vi "Teleop.vi"(10 "Match Info":T1={"Autonomous Elapsed Seconds"=0.0, "TeleOp Elapsed Seconds"=0.0, "Disabled Elapsed Seconds"=0.0, "Visited Autonomous"=FALSE, "Visited TeleOp"=FALSE, "Visited Disabled"=FALSE, "Autonomous Settings"={"Autonomous Style"=enum."Independent", "VI Refnum"=refnum}}, 11 "Call Context":T2) -> ()   [LabVIEW 2020]
doc: "This VI is called for each TeleOp packet received from the DS where the robot is not disabled. It is often used to read from the joysticks and update I/O or to update setpoints for timed control loops. It should complete and return within 20 milliseconds or it may miss DS packets."
uses:
  <vilib>/Rock Robotics/WPI/DriverStation/WPI_DriverStationDerivedRobotMode.ctl
  <vilib>/Rock Robotics/WPI/DriverStation/WPI_DriverStationMatch Info.ctl
  <vilib>/Rock Robotics/WPI/ThirdParty/Phoenix-LabVIEW/Motor Controller/Controls/CTRE_Phoenix_MotorControl_ControlMode.ctl
  <vilib>/Rock Robotics/Network Tables/NT Read Boolean.vi
  GlobalVariables.vi
  <vilib>/Rock Robotics/Network Tables/NT Read Number.vi
panel:
  out "Rate_Add":dbl
  out "Stop_pid":bool=TRUE
  out "Corrente total":dbl
  out "Sample Slider 0":dbl(slide) scale=0.0..5.0
  out "Sample Boolean 1":bool
  out "Sample Boolean 0":bool
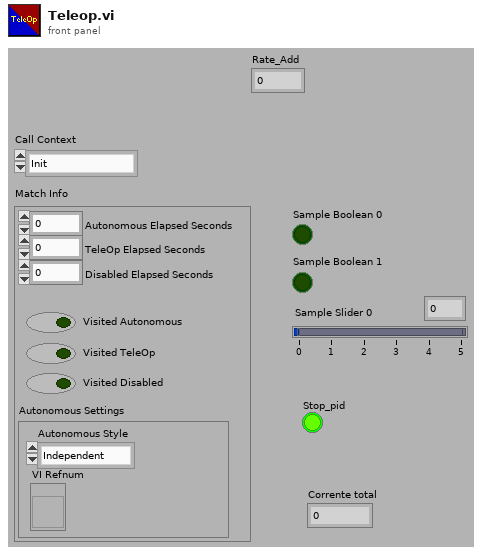
[diagram p1: front panel]
types:
  T1 = typedef "WPI_DriverStationMatch Info.ctl" = cluster{"Autonomous Elapsed Seconds":dbl, "TeleOp Elapsed Seconds":dbl, "Disabled Elapsed Seconds":dbl, "Visited Autonomous":bool, "Visited TeleOp":bool, "Visited Disabled":bool, "Autonomous Settings":cluster{"Autonomous Style":enum16{"Iterative", "Independent"}, "VI Refnum":refnum<vi>}}
  T2 = typedef "WPI_DriverStationDerivedRobotMode.ctl" = enum16{"Init", "Execute", "Stop"}
  T3 = typedef "CTRE_Phoenix_MotorControl_ControlMode.ctl" = u16
  T4 = typedef "WPI_MotorControlDeviceRef.ctl" = cluster{"DeviceStatus":errorcluster, "Type":T5, "PWM":cluster{"PWM Channel":T6, "DeadBand":T7}, "CAN":cluster{"Device Number":u8, "SetOutput VI Ref":variant, "GetOutput VI Ref":variant, "Enable VI Ref":variant, "Disable VI Ref":variant, "Data":variant}, "Invert":bool, "DIO PWM":cluster{"PWM \"Enable\" Channel":T6, "DIOChannel":T8, "PWM Rate":dbl}}
  T5 = typedef "WPI_MotorControlType.ctl" = enum16{"PWM", "CAN", "DIO PWM"}
  T6 = typedef "FPGA_DIOPWMChannel.ctl" = enum8{"PWM 0", "PWM 1", "PWM 2", "PWM 3", "PWM 4", "PWM 5", "PWM 6", "PWM 7", "PWM 8", "PWM 9", "PWM MXP 0", "PWM MXP 1", "PWM MXP 2", "PWM MXP 3", "PWM MXP 4", "PWM MXP 5", "PWM MXP 6", "PWM MXP 7", "PWM MXP 8", "PWM MXP 9", "Invalid"}
  T7 = typedef "WPI_PWMDeadband.ctl" = cluster{"Name":string, "maxPositivePwm":i32, "minPositivePwm":i32, "centerPwm":i32, "maxNegativePwm":i32, "minNegativePwm":i32, "angularRange":u16}
  T8 = typedef "FPGA_DIOChannel.ctl" = enum8{"DIO 0", "DIO 1", "DIO 2", "DIO 3", "DIO 4", "DIO 5", "DIO 6", "DIO 7", "DIO 8", "DIO 9", "DIO MXP 0", "DIO MXP 1", "DIO MXP 2", "DIO MXP 3", "DIO MXP 4", "DIO MXP 5", "DIO MXP 6", "DIO MXP 7", "DIO MXP 8", "DIO MXP 9", "DIO MXP 10", "DIO MXP 11", "DIO MXP 12", "DIO MXP 13", "DIO MXP 14", "DIO MXP 15", "SPI Port CS1", "SPI Port CS2", "SPI Port CS3", "SPI Port MISO", "SPI Port MOSI", "Invalid"}
  T9 = cluster{"Buttons[0]":bool, "Buttons[1]":bool, "Buttons[2]":bool, "Buttons[3]":bool, "Buttons[4]":bool, "Buttons[5]":bool, "Buttons[6]":bool, "Buttons[7]":bool, "Buttons[8]":bool, "Buttons[9]":bool}
  T10 = cluster{"Axes[0]":dbl, "Axes[1]":dbl, "Axes[2]":dbl, "Axes[3]":dbl, "Axes[4]":dbl, "Axes[5]":dbl, "Axes[6]":dbl, "Axes[7]":dbl}
  T11 = cluster{"Axes[0]":dbl, "Axes[1]":dbl, "Axes[2]":dbl, "Axes[3]":dbl}
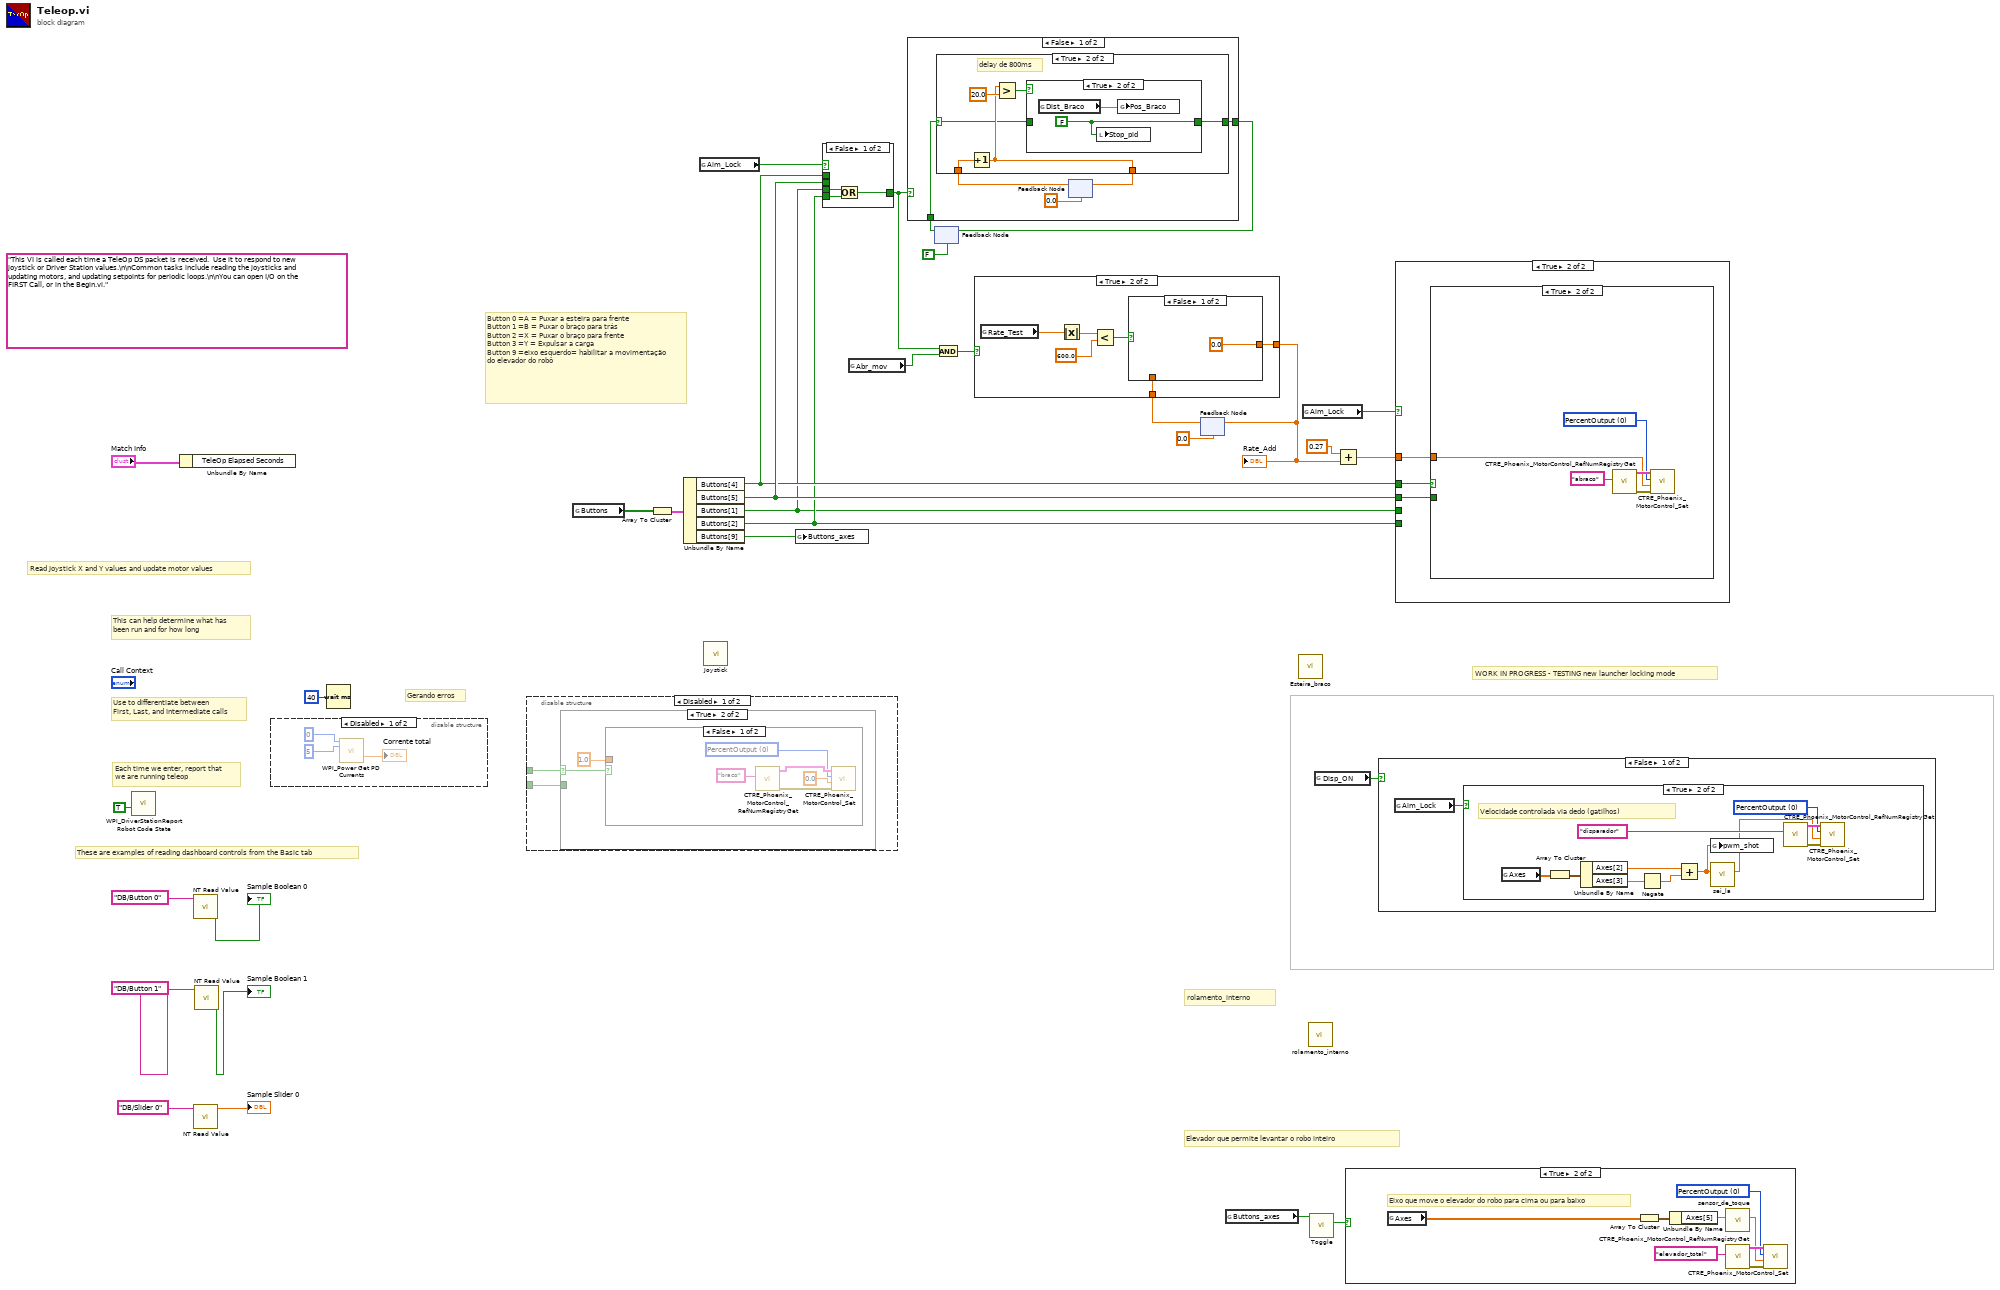
[diagram p0: block diagram]
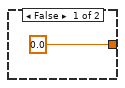
[diagram p2: hidden frame]
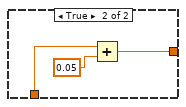
[diagram p3: hidden frame]
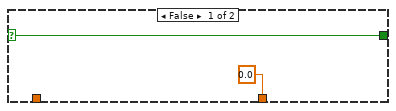
[diagram p4: hidden frame]
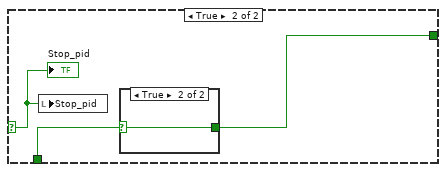
[diagram p6: hidden frame]
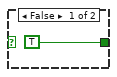
[diagram p7: hidden frame]
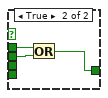
[diagram p8: hidden frame]
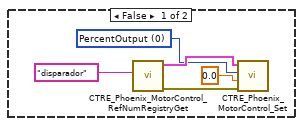
[diagram p9: hidden frame]
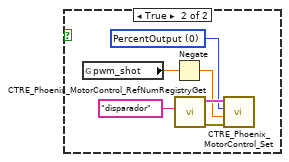
[diagram p10: hidden frame]
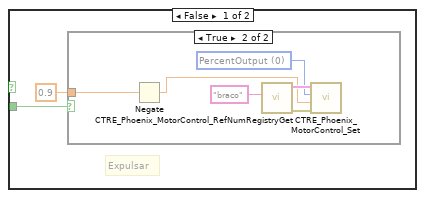
[diagram p12: hidden frame]
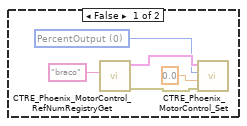
[diagram p13: hidden frame]
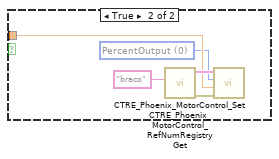
[diagram p14: hidden frame]
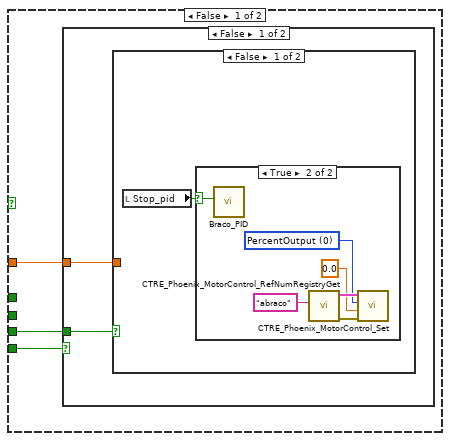
[diagram p16: hidden frame]
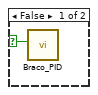
[diagram p17: hidden frame]
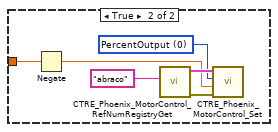
[diagram p18: hidden frame]
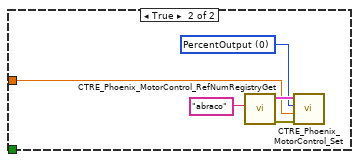
[diagram p19: hidden frame]
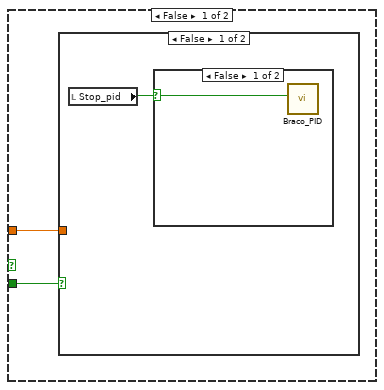
[diagram p20: hidden frame]
diagram:
  (unwired) "This VI is called each time a TeleOp DS packet is received.  Use it to respond to new joystick or Driver Station values.\n\nCommon tasks include reading the joysticks and updating motors, and updating setpoints for periodic loops.\n\nYou can open I/O on the FIRST Call, or in the Begin.vi."
  # "WORK IN PROGRESS - TESTING new launcher locking mode"
  # "Gerando erros"
  # "rolamento_interno"
  # "Elevador que permite levantar o robo inteiro"
  # "Button 0 =A = Puxar a esteira para frente  \nButton 1 =B = Puxar o braço para trás \nButton 2 =X = Puxar o braço para frente  \nButton 3 =Y = Expulsar a carga\nButton 9 =eixo esquerdo= habilitar a movimentação do elevador do robô"
  # "These are examples of reading dashboard controls from the Basic tab"
  # "Each time we enter, report that\nwe are running teleop"
  # "Use to differentiate between\nFirst, Last, and Intermediate calls"
  # "This can help determine what has\nbeen run and for how long"
  # "Read Joystick X and Y values and update motor values"
  n1 = call <vilib>:"WPI_DriverStationReport Robot Code State.vi"("TeleOp"=TRUE ("Autonomous")) -> ()  [unwired: 10 in, 1 out]
  n2 = Unbundle By Name("Match Info") -> ()  [unwired: 1 out]
  n3 = call-poly <vilib>:"NT Read Value.vi"("Name"="DB/Button 0" ("refnum name")) -> ("Boolean"=→"Sample Boolean 0":bool)  [unwired: 9 in, 1 out]
  n4 = call-poly <vilib>:"NT Read Value.vi"("Name"="DB/Slider 0" ("refnum name")) -> ("Numeric"=→"Sample Slider 0":dbl)  [unwired: 9 in, 1 out]
  n5 = call-poly <vilib>:"NT Read Value.vi"("Name"="DB/Button 1" ("refnum name")) -> ("Boolean"=→"Sample Boolean 1":bool)  [unwired: 9 in, 1 out]
  n6 = disable-structure shown="Disabled" {
    frame Disabled {
      n7 = call <vilib>:"WPI_Power Get PD Currents.vi"("Power Distribution (def)"=u8 0, "PD Channel"=5) -> ("total current (A)"=→"Corrente total":dbl)  [unwired: 10 in, 3 out]
    }
    frame Enabled {
    }
  }
  n8 = Wait (ms)(milliseconds to wait=40) -> ()  [unwired: 1 out]
  n9 = disable-structure shown="Disabled" {
    disable-tunnel: _ -> [w37 _]
    disable-tunnel: _ -> [w36 _]
    frame Disabled {
      n10 = case shown="True" w36 {
        selector: w36 -> [_ w52]
        tunnel: w37 -> [w38 _]
        frame False {
          # "Expulsar"
          n11 = case shown="True" w38 {
            tunnel: 0.9 -> [_ w46]
            frame False {
              w41 = T3 0 items=["PercentOutput"=0, "Position"=1, "Velocity"=2, "Current"=3, "Follower"=5, "MotionProfile"=6, "MotionMagic"=7, "MotionProfileArc"=10, "Disabled"=15] ("Control Mode")
              n12 = call <vilib>:"CTRE_Phoenix_MotorControl_RefNumRegistryGet.vi"("refnum name"="braco") -> ("error out"=w44:errorcluster, "PhoenixMotorControlDevRef"=w43:T4)  [unwired: 9 in]
              n13 = call <vilib>:"CTRE_Phoenix_MotorControl_Set.vi"("error in (no error)"=w44, "Output"=0.0, "Control Mode"=w41, "PhoenixMotorControlDevRef"=w43) -> ()  [unwired: 6 in, 2 out]
            }
            frame True {
              w48 = T3 0 items=["PercentOutput"=0, "Position"=1, "Velocity"=2, "Current"=3, "Follower"=5, "MotionProfile"=6, "MotionMagic"=7, "MotionProfileArc"=10, "Disabled"=15] ("Control Mode")
              n14 = Negate(x=w46) -> (-x=w45:dbl)
              n15 = call <vilib>:"CTRE_Phoenix_MotorControl_RefNumRegistryGet.vi"("refnum name"="braco") -> ("error out"=w49:errorcluster, "PhoenixMotorControlDevRef"=w50:T4)  [unwired: 9 in]
              n16 = call <vilib>:"CTRE_Phoenix_MotorControl_Set.vi"("error in (no error)"=w49, "Output"=w45, "Control Mode"=w48, "PhoenixMotorControlDevRef"=w50) -> ()  [unwired: 6 in, 2 out]
            }
          }
        }
        frame True {
          n17 = case shown="False" w52 {
            tunnel: 1.0 ("Output") -> [_ w60]
            frame False {
              w54 = T3 0 items=["PercentOutput"=0, "Position"=1, "Velocity"=2, "Current"=3, "Follower"=5, "MotionProfile"=6, "MotionMagic"=7, "MotionProfileArc"=10, "Disabled"=15] ("Control Mode")
              n18 = call <vilib>:"CTRE_Phoenix_MotorControl_RefNumRegistryGet.vi"("refnum name"="braco") -> ("error out"=w57:errorcluster, "PhoenixMotorControlDevRef"=w56:T4)  [unwired: 9 in]
              n19 = call <vilib>:"CTRE_Phoenix_MotorControl_Set.vi"("error in (no error)"=w57, "Output"=0.0, "Control Mode"=w54, "PhoenixMotorControlDevRef"=w56) -> ()  [unwired: 6 in, 2 out]
            }
            frame True {
              w59 = T3 0 items=["PercentOutput"=0, "Position"=1, "Velocity"=2, "Current"=3, "Follower"=5, "MotionProfile"=6, "MotionMagic"=7, "MotionProfileArc"=10, "Disabled"=15] ("Control Mode")
              n20 = call <vilib>:"CTRE_Phoenix_MotorControl_RefNumRegistryGet.vi"("refnum name"="braco") -> ("error out"=w61:errorcluster, "PhoenixMotorControlDevRef"=w62:T4)  [unwired: 9 in]
              n21 = call <vilib>:"CTRE_Phoenix_MotorControl_Set.vi"("error in (no error)"=w61, "Output"=w60, "Control Mode"=w59, "PhoenixMotorControlDevRef"=w62) -> ()  [unwired: 6 in, 2 out]
            }
          }
        }
      }
    }
    frame Enabled {
    }
  }
  n22 = global read "GlobalVariables.vi" "Buttons"() -> (w21:bool[])
  n23 = Array To Cluster(array=w21) -> (cluster=w22:T9)
  n24 = Unbundle By Name(w22) -> ("Buttons[4]"=w17:bool, "Buttons[5]"=w18:bool, "Buttons[1]"=w15:bool, "Buttons[2]"=w16:bool, "Buttons[9]"=w9:bool)
  n25 = global read "GlobalVariables.vi" "Aim_Lock"() -> (w10:bool)
  n26 = call "Joystick.vi"() -> ()  [unwired: 11 in]
  n27 = global write "GlobalVariables.vi" "Buttons_axes"(w9) -> ()
  n28 = case shown="False" w10 {
    tunnel: w18 -> [_ w68]
    tunnel: w17 -> [_ w67]
    tunnel: w16 -> [w65 _]
    tunnel: w15 -> [w64 _]
    tunnel: [w63 w66] -> w8
    frame False {
      n29 = Or(x=w64, y=w65) -> (x .or. y?=w63:bool)
    }
    frame True {
      n30 = Or(x=w67, y=w68) -> (x .or. y?=w66:bool)
    }
  }
  n31 = global read "GlobalVariables.vi" "Abr_mov"() -> (w7:bool)
  n32 = feedback #1(FALSE) -> (w12:bool)
  n33 = case shown="False" w8 {
    selector: w8 -> [_ w85]
    tunnel: w12 -> [w72 w87]
    tunnel: [w73 w86] -> w11
    frame False {
      n34 = feedback #2(0.0) -> (w69:dbl)
      n35 = case shown="True" w72 {
        selector: w72 -> [w75 w76]
        tunnel: [w75 w81] -> w73
        tunnel: [0.0 w77] -> w70
        tunnel: w69 -> [_ w78]
        frame False {
        }
        frame True {
          # "delay de 800ms"
          n36 = Increment(x=w78) -> (x+1=w77:dbl)
          n37 = Greater?(x=w77, y=20.0) -> (0:w80:bool)
          n38 = case shown="True" w80 {
            tunnel: [w82 w83] -> w81
            tunnel: w76 -> [w82 _]
            frame False {
            }
            frame True {
              w83 = FALSE
              n39 = global read "GlobalVariables.vi" "Dist_Braco"() -> (w84:dbl)
              n40 = local write "Stop_pid"(w83) -> ()
              n41 = global write "GlobalVariables.vi" "Pos_Braco"(w84) -> ()
            }
          }
        }
      }
      n42 = feedback-in #2(w70) -> ()
    }
    frame True {
      n43 = local write "Stop_pid"(w85) -> ()
      n44 = case shown="True" w87 {
        selector: w87 -> [_ w89]
        tunnel: [TRUE w89] -> w86
        frame False {
        }
        frame True {
        }
      }
      "Stop_pid" <- w85
    }
  }
  n45 = feedback-in #1(w11) -> ()
  n46 = And(x=w8, y=w7) -> (x .and. y?=w6:bool)
  n47 = feedback #3(0.0) -> (w4:dbl)
  n48 = case shown="True" w6 {
    tunnel: w4 -> [_ w92]
    tunnel: [0.0 w91] -> w3
    frame False {
    }
    frame True {
      n49 = global read "GlobalVariables.vi" "Rate_Test"() -> (w96:dbl)
      n50 = Absolute Value(x=w96) -> (abs(x)=w95:dbl)
      n51 = Less?(x=w95, y=600.0) -> (x < y?=w93:bool)
      n52 = case shown="False" w93 {
        tunnel: w92 -> [_ w99]
        tunnel: [0.0 w98] -> w91
        frame False {
        }
        frame True {
          n53 = Add(x=w99, y=0.05) -> (x+y=w98:dbl)
        }
      }
    }
  }
  "Rate_Add" <- w3
  n54 = feedback-in #3(w3) -> ()
  n55 = global read "GlobalVariables.vi" "Buttons_axes"() -> (w19:bool)
  n56 = call "Esteira_braco.vi"() -> ()  [unwired: 12 in]
  n57 = global read "GlobalVariables.vi" "Aim_Lock"() -> (w20:bool)
  n58 = call "rolamento_interno.vi"() -> ()  [unwired: 12 in]
  n59 = call "Toggle.vi"("Input"=w19) -> ("Output"=w23:bool)  [unwired: 10 in]
  n60 = global read "GlobalVariables.vi" "Disp_ON"() -> (w14:bool)
  n61 = Add(x=0.27, y=w3) -> (x+y=w1:dbl)
  n62 = case shown="True" w23 {
    frame False {
      w104 = T3 0 items=["PercentOutput"=0, "Position"=1, "Velocity"=2, "Current"=3, "Follower"=5, "MotionProfile"=6, "MotionMagic"=7, "MotionProfileArc"=10, "Disabled"=15] ("Control Mode")
      n63 = call <vilib>:"CTRE_Phoenix_MotorControl_RefNumRegistryGet.vi"("refnum name"="elevador_total") -> ("error out"=w103:errorcluster, "PhoenixMotorControlDevRef"=w102:T4)  [unwired: 9 in]
      n64 = call <vilib>:"CTRE_Phoenix_MotorControl_Set.vi"("error in (no error)"=w103, "Output"=0.0, "Control Mode"=w104, "PhoenixMotorControlDevRef"=w102) -> ()  [unwired: 6 in, 2 out]
    }
    frame True {
      w110 = T3 0 items=["PercentOutput"=0, "Position"=1, "Velocity"=2, "Current"=3, "Follower"=5, "MotionProfile"=6, "MotionMagic"=7, "MotionProfileArc"=10, "Disabled"=15] ("Control Mode")
      # "Eixo que move o elevador do robo para cima ou para baixo"
      n65 = global read "GlobalVariables.vi" "Axes"() -> (w108:dbl[])
      n66 = Array To Cluster(array=w108) -> (cluster=w113:T10)
      n67 = Unbundle By Name(w113) -> ("Axes[5]"=w107:dbl)
      n68 = call "sensor_de_toque.vi"("valor_eixo"=w107) -> ("parada"=w106:dbl)  [unwired: 9 in]
      n69 = call <vilib>:"CTRE_Phoenix_MotorControl_RefNumRegistryGet.vi"("refnum name"="elevador_total") -> ("error out"=w112:errorcluster, "PhoenixMotorControlDevRef"=w111:T4)  [unwired: 9 in]
      n70 = call <vilib>:"CTRE_Phoenix_MotorControl_Set.vi"("error in (no error)"=w112, "Output"=w106, "Control Mode"=w110, "PhoenixMotorControlDevRef"=w111) -> ()  [unwired: 6 in, 2 out]
    }
  }
  n71 = case shown="False" w14 {
    frame False {
      n72 = global read "GlobalVariables.vi" "Aim_Lock"() -> (w114:bool)
      n73 = case shown="True" w114 {
        frame False {
          w116 = T3 0 items=["PercentOutput"=0, "Position"=1, "Velocity"=2, "Current"=3, "Follower"=5, "MotionProfile"=6, "MotionMagic"=7, "MotionProfileArc"=10, "Disabled"=15] ("Control Mode")
          n74 = call <vilib>:"CTRE_Phoenix_MotorControl_RefNumRegistryGet.vi"("refnum name"="disparador") -> ("error out"=w117:errorcluster, "PhoenixMotorControlDevRef"=w118:T4)  [unwired: 9 in]
          n75 = call <vilib>:"CTRE_Phoenix_MotorControl_Set.vi"("error in (no error)"=w117, "Output"=0.0, "Control Mode"=w116, "PhoenixMotorControlDevRef"=w118) -> ()  [unwired: 6 in, 2 out]
        }
        frame True {
          w127 = T3 0 items=["PercentOutput"=0, "Position"=1, "Velocity"=2, "Current"=3, "Follower"=5, "MotionProfile"=6, "MotionMagic"=7, "MotionProfileArc"=10, "Disabled"=15] ("Control Mode")
          # "Velocidade controlada via dedo (gatilhos)"
          n76 = global read "GlobalVariables.vi" "Axes"() -> (w121:dbl[])
          n77 = Array To Cluster(array=w121) -> (cluster=w130:T11)
          n78 = Unbundle By Name(w130) -> ("Axes[2]"=w123:dbl, "Axes[3]"=w124:dbl)
          n79 = Negate(x=w124) -> (-x=w125:dbl)
          n80 = Add(x=w123, y=w125) -> (x+y=w120:dbl)
          n81 = global write "GlobalVariables.vi" "pwm_shot"(w120) -> ()
          n82 = call "sei_la.vi"("INPUT"=w120) -> ("Output"=w122:dbl)  [unwired: 10 in]
          n83 = call <vilib>:"CTRE_Phoenix_MotorControl_RefNumRegistryGet.vi"("refnum name"="disparador") -> ("error out"=w126:errorcluster, "PhoenixMotorControlDevRef"=w128:T4)  [unwired: 9 in]
          n84 = call <vilib>:"CTRE_Phoenix_MotorControl_Set.vi"("error in (no error)"=w126, "Output"=w122, "Control Mode"=w127, "PhoenixMotorControlDevRef"=w128) -> ()  [unwired: 6 in, 2 out]
        }
      }
    }
    frame True {
      w133 = T3 0 items=["PercentOutput"=0, "Position"=1, "Velocity"=2, "Current"=3, "Follower"=5, "MotionProfile"=6, "MotionMagic"=7, "MotionProfileArc"=10, "Disabled"=15] ("Control Mode")
      n85 = global read "GlobalVariables.vi" "pwm_shot"() -> (w131:dbl)
      n86 = Negate(x=w131) -> (-x=w132:dbl)
      n87 = call <vilib>:"CTRE_Phoenix_MotorControl_RefNumRegistryGet.vi"("refnum name"="disparador") -> ("error out"=w134:errorcluster, "PhoenixMotorControlDevRef"=w135:T4)  [unwired: 9 in]
      n88 = call <vilib>:"CTRE_Phoenix_MotorControl_Set.vi"("error in (no error)"=w134, "Output"=w132, "Control Mode"=w133, "PhoenixMotorControlDevRef"=w135) -> ()  [unwired: 6 in, 2 out]
    }
  }
  n89 = case shown="True" w20 {
    tunnel: w15 -> [w138 _]
    tunnel: w16 -> [w139 _]
    tunnel: w17 -> [_ w163]
    tunnel: w18 -> [_ w162]
    tunnel: w1 -> [w137 w161]
    frame False {
      n90 = case shown="False" w139 {
        tunnel: w138 -> [w141 _]
        tunnel: w137 -> [w140 w156]
        frame False {
          n91 = case shown="False" w141 {
            tunnel: w140 -> [_ w155]
            frame False {
              n92 = local read "Stop_pid"() -> (w142:bool)
              n93 = case shown="True" w142 {
                selector: w142 -> [w143 w149]
                frame False {
                  n94 = call "Braco_PID.vi"("Stop_PID"=w143) -> ()  [unwired: 11 in]
                }
                frame True {
                  w145 = T3 0 items=["PercentOutput"=0, "Position"=1, "Velocity"=2, "Current"=3, "Follower"=5, "MotionProfile"=6, "MotionMagic"=7, "MotionProfileArc"=10, "Disabled"=15] ("Control Mode")
                  n95 = call "Braco_PID.vi"("Stop_PID"=w149) -> ()  [unwired: 11 in]
                  n96 = call <vilib>:"CTRE_Phoenix_MotorControl_RefNumRegistryGet.vi"("refnum name"="abraco") -> ("error out"=w148:errorcluster, "PhoenixMotorControlDevRef"=w147:T4)  [unwired: 9 in]
                  n97 = call <vilib>:"CTRE_Phoenix_MotorControl_Set.vi"("error in (no error)"=w148, "Output"=0.0, "Control Mode"=w145, "PhoenixMotorControlDevRef"=w147) -> ()  [unwired: 6 in, 2 out]
                }
              }
            }
            frame True {
              w151 = T3 0 items=["PercentOutput"=0, "Position"=1, "Velocity"=2, "Current"=3, "Follower"=5, "MotionProfile"=6, "MotionMagic"=7, "MotionProfileArc"=10, "Disabled"=15] ("Control Mode")
              n98 = Negate(x=w155) -> (-x=w150:dbl)
              n99 = call <vilib>:"CTRE_Phoenix_MotorControl_RefNumRegistryGet.vi"("refnum name"="abraco") -> ("error out"=w153:errorcluster, "PhoenixMotorControlDevRef"=w152:T4)  [unwired: 9 in]
              n100 = call <vilib>:"CTRE_Phoenix_MotorControl_Set.vi"("error in (no error)"=w153, "Output"=w150, "Control Mode"=w151, "PhoenixMotorControlDevRef"=w152) -> ()  [unwired: 6 in, 2 out]
            }
          }
        }
        frame True {
          w157 = T3 0 items=["PercentOutput"=0, "Position"=1, "Velocity"=2, "Current"=3, "Follower"=5, "MotionProfile"=6, "MotionMagic"=7, "MotionProfileArc"=10, "Disabled"=15] ("Control Mode")
          n101 = call <vilib>:"CTRE_Phoenix_MotorControl_RefNumRegistryGet.vi"("refnum name"="abraco") -> ("error out"=w159:errorcluster, "PhoenixMotorControlDevRef"=w160:T4)  [unwired: 9 in]
          n102 = call <vilib>:"CTRE_Phoenix_MotorControl_Set.vi"("error in (no error)"=w159, "Output"=w156, "Control Mode"=w157, "PhoenixMotorControlDevRef"=w160) -> ()  [unwired: 6 in, 2 out]
        }
      }
    }
    frame True {
      n103 = case shown="True" w163 {
        tunnel: w162 -> [w165 _]
        tunnel: w161 -> [w164 w180]
        frame False {
          n104 = case shown="False" w165 {
            tunnel: w164 -> [_ w174]
            frame False {
              n105 = local read "Stop_pid"() -> (w166:bool)
              n106 = case shown="False" w166 {
                selector: w166 -> [w167 w173]
                frame False {
                  n107 = call "Braco_PID.vi"("Stop_PID"=w167) -> ()  [unwired: 11 in]
                }
                frame True {
                  w169 = T3 0 items=["PercentOutput"=0, "Position"=1, "Velocity"=2, "Current"=3, "Follower"=5, "MotionProfile"=6, "MotionMagic"=7, "MotionProfileArc"=10, "Disabled"=15] ("Control Mode")
                  n108 = call "Braco_PID.vi"("Stop_PID"=w173) -> ()  [unwired: 11 in]
                  n109 = call <vilib>:"CTRE_Phoenix_MotorControl_RefNumRegistryGet.vi"("refnum name"="abraco") -> ("error out"=w172:errorcluster, "PhoenixMotorControlDevRef"=w171:T4)  [unwired: 9 in]
                  n110 = call <vilib>:"CTRE_Phoenix_MotorControl_Set.vi"("error in (no error)"=w172, "Output"=0.0, "Control Mode"=w169, "PhoenixMotorControlDevRef"=w171) -> ()  [unwired: 6 in, 2 out]
                }
              }
            }
            frame True {
              w176 = T3 0 items=["PercentOutput"=0, "Position"=1, "Velocity"=2, "Current"=3, "Follower"=5, "MotionProfile"=6, "MotionMagic"=7, "MotionProfileArc"=10, "Disabled"=15] ("Control Mode")
              n111 = Negate(x=w174) -> (-x=w175:dbl)
              n112 = call <vilib>:"CTRE_Phoenix_MotorControl_RefNumRegistryGet.vi"("refnum name"="abraco") -> ("error out"=w178:errorcluster, "PhoenixMotorControlDevRef"=w177:T4)  [unwired: 9 in]
              n113 = call <vilib>:"CTRE_Phoenix_MotorControl_Set.vi"("error in (no error)"=w178, "Output"=w175, "Control Mode"=w176, "PhoenixMotorControlDevRef"=w177) -> ()  [unwired: 6 in, 2 out]
            }
          }
        }
        frame True {
          w181 = T3 0 items=["PercentOutput"=0, "Position"=1, "Velocity"=2, "Current"=3, "Follower"=5, "MotionProfile"=6, "MotionMagic"=7, "MotionProfileArc"=10, "Disabled"=15] ("Control Mode")
          n114 = call <vilib>:"CTRE_Phoenix_MotorControl_RefNumRegistryGet.vi"("refnum name"="abraco") -> ("error out"=w183:errorcluster, "PhoenixMotorControlDevRef"=w184:T4)  [unwired: 9 in]
          n115 = call <vilib>:"CTRE_Phoenix_MotorControl_Set.vi"("error in (no error)"=w183, "Output"=w180, "Control Mode"=w181, "PhoenixMotorControlDevRef"=w184) -> ()  [unwired: 6 in, 2 out]
        }
      }
    }
  }
